vi "Memory.Pointer.Error Handling.Write Range to Error.vi"(7 "parameter":T1, 8 "value":u64, 9 "offset":i32, 10 "error in":errorcluster, 11 "Pointer in":refnum<class "Memory.Pointer.lvclass">) -> (1 "new offset":i32, 2 "error out":errorcluster, 3 "Pointer out":refnum<class "Memory.Pointer.lvclass">)   [LabVIEW 2016, in "LabVIEW Memory Manager.lvlib" / "Memory.Pointer.lvclass"]
uses:
  Memory.Pointer.lvclass
  Typedefs/Memory.Pointer.Parameters.ctl
  Memory.Pointer.lvclass/Memory.Pointer.ctl
  RT Errors/Deterministic Errors.lvlib
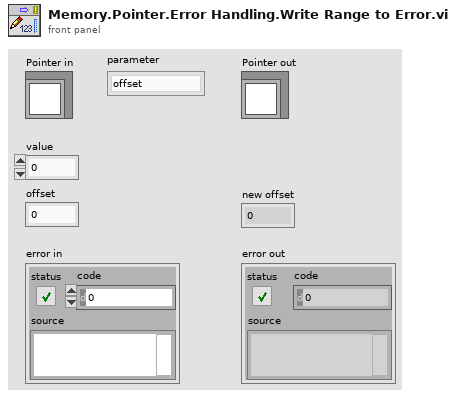
[diagram p1: front panel]
types:
  T1 = typedef "LabVIEW Memory Manager.lvlib/Memory.Pointer.lvclass/Memory.Pointer.Parameters.ctl" = enum16{"offset", "length", "size", "subset"}
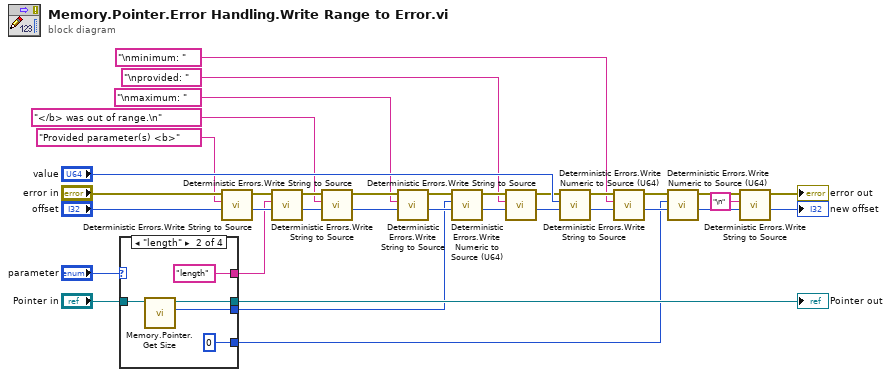
[diagram p0: block diagram]
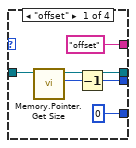
[diagram p2: hidden frame]
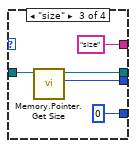
[diagram p3: hidden frame]
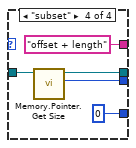
[diagram p4: hidden frame]
diagram:
  n1 = case shown="\"length\"" "parameter" {
    tunnel: "Pointer in" -> [w40 w45 w50 w55]
    tunnel: ["offset" "length" "size" "offset + length"] -> w5
    tunnel: [w36 w44 w49 w54] -> w1
    tunnel: [w38 w43 w48 w53] -> w29
    tunnel: [u64 0 ("size") u64 0 ("size") u64 0 ("size") u64 0 ("size")] -> w2
    frame "offset" {
      n2 = call "Memory.Pointer.Get Size.vi"("Pointer in"=w40) -> ("size"=w39:u64, "Pointer out"=w38:refnum<class "Memory.Pointer.lvclass">)  [unwired: 8 in, 1 out]
      n3 = Decrement(x=w39) -> (x-1=w36:u64)
    }
    frame "length" {
      n4 = call "Memory.Pointer.Get Size.vi"("Pointer in"=w45) -> ("size"=w44:u64, "Pointer out"=w43:refnum<class "Memory.Pointer.lvclass">)  [unwired: 8 in, 1 out]
    }
    frame "size" {
      n5 = call "Memory.Pointer.Get Size.vi"("Pointer in"=w50) -> ("size"=w49:u64, "Pointer out"=w48:refnum<class "Memory.Pointer.lvclass">)  [unwired: 8 in, 1 out]
    }
    frame "subset" {
      n6 = call "Memory.Pointer.Get Size.vi"("Pointer in"=w55) -> ("size"=w54:u64, "Pointer out"=w53:refnum<class "Memory.Pointer.lvclass">)  [unwired: 8 in, 1 out]
    }
  }
  "Pointer out" <- w29
  n7 = call "Deterministic Errors.Write String to Source.vi"("offset (0)"="offset", "string"="Provided parameter(s) <b>", "error in"="error in") -> ("new offset"=w10:i32, "error out"=w12:errorcluster)  [unwired: 7 in]
  n8 = call "Deterministic Errors.Write String to Source.vi"("offset (0)"=w10, "string"=w5, "error in"=w12) -> ("new offset"=w9:i32, "error out"=w11:errorcluster)  [unwired: 7 in]
  n9 = call "Deterministic Errors.Write String to Source.vi"("offset (0)"=w9, "string"="</b> was out of range.\n", "error in"=w11) -> ("new offset"=w8:i32, "error out"=w7:errorcluster)  [unwired: 7 in]
  n10 = call "Deterministic Errors.Write String to Source.vi"("offset (0)"=w8, "string"="\nmaximum: ", "error in"=w7) -> ("new offset"=w24:i32, "error out"=w27:errorcluster)  [unwired: 7 in]
  n11 = call "Deterministic Errors.Write Numeric to Source (U64).vi"("offset (0)"=w24, "value"=w1, "error in"=w27) -> ("new offset"=w25:i32, "error out"=w26:errorcluster)  [unwired: 7 in]
  n12 = call "Deterministic Errors.Write String to Source.vi"("offset (0)"=w25, "string"="\nprovided: ", "error in"=w26) -> ("new offset"=w21:i32, "error out"=w22:errorcluster)  [unwired: 7 in]
  n13 = call "Deterministic Errors.Write Numeric to Source (U64).vi"("offset (0)"=w21, "value"="value", "error in"=w22) -> ("new offset"=w19:i32, "error out"=w20:errorcluster)  [unwired: 7 in]
  n14 = call "Deterministic Errors.Write String to Source.vi"("offset (0)"=w19, "string"="\nminimum: ", "error in"=w20) -> ("new offset"=w17:i32, "error out"=w18:errorcluster)  [unwired: 7 in]
  n15 = call "Deterministic Errors.Write Numeric to Source (U64).vi"("offset (0)"=w17, "value"=w2, "error in"=w18) -> ("new offset"=w14:i32, "error out"=w16:errorcluster)  [unwired: 7 in]
  n16 = call "Deterministic Errors.Write String to Source.vi"("offset (0)"=w14, "string"="\n", "error in"=w16) -> ("new offset"=→"new offset":i32, "error out"=→"error out":errorcluster)  [unwired: 7 in]
